vi "Read CAN FIFO Direct Dispatch.vi"(8 "error in (no error)":errorcluster, 9 "Timeout (ms)":i32, 11 "CIFTag in":refnum<class "CIFChannels.lvclass">) -> (0 "error out":errorcluster, 1 "timed out?":bool, 2 "Data":T1[](array[typedef]) {"Tags" format="%.0x"; "payload" format="%x"; "identifier" format="%x"}, 3 "CIFTag out":refnum<class "CIF_NIChn_FifoCAN.lvclass">, 4 "Header":T2)   [LabVIEW 2021, in "CIF_NIChn_FifoCAN.lvclass"]
uses:
  CIF_NIChn_FifoCAN.lvclass
  CIF_NIChn_FifoCAN.lvclass/CIF_NIChn_FifoCAN.ctl
  CIFChannels/Typedef/Direction.ctl
  CIFChannels/CIFChannels.lvclass
  CIFChannels/Typedef/Channel State.ctl
  NIChn/CIF_NIChn.lvclass
  D:/dev/CIF-LVCore/src/Channels/CIF_NIChn/NIChn/CIF_NIChn.lvclass
  D:/dev/CIF-LVCore/src/Channels/CIFChannels/CIFChannels.lvclass
  D:/dev/CIF-LVCore/src/Channels/CIF_NIChn/FIFO_CAN/CIF_NIChn_FifoCAN.lvclass
  <vilib>/CIFChannels/CIFChannelCore.lvlib
  ChannelRegistrar/typedef/Datatype CAN.ctl
  ChannelRegistrar/ChannelRegistrar.lvlib
  ChannelCommon/typedef/FIFO Header.ctl
  ChannelCommon/ChannelCommon.lvlib
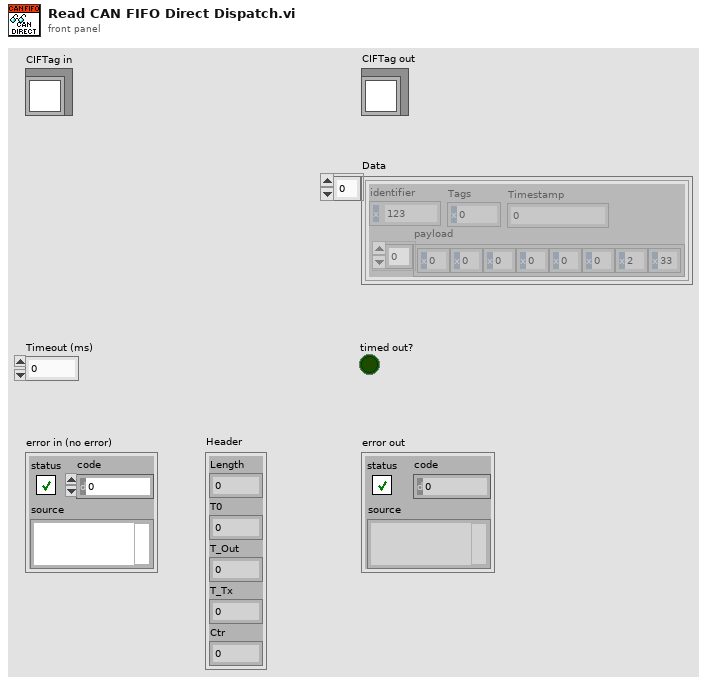
[diagram p1: front panel]
types:
  T1 = typedef "ChannelRegistrar.lvlib/Datatype CAN.ctl" = cluster{"payload":u8[], "identifier":u32, "Tags":u8, "Timestamp":u64}
  T2 = typedef "ChannelCommon.lvlib/FIFO Header.ctl" = cluster{"Length":u64, "T0":u64, "T_Out":u64, "T_Tx":u64, "Ctr":u64}
  T3 = typedef "CIFChannels.lvclass/Channel State.ctl" = enum16{"Creating", "Disconnected", "Connecting", "Connected", "Destroyed"}
  T4 = typedef "CIFChannels.lvclass/Direction.ctl" = enum16{"Publisher", "Subscriber"}
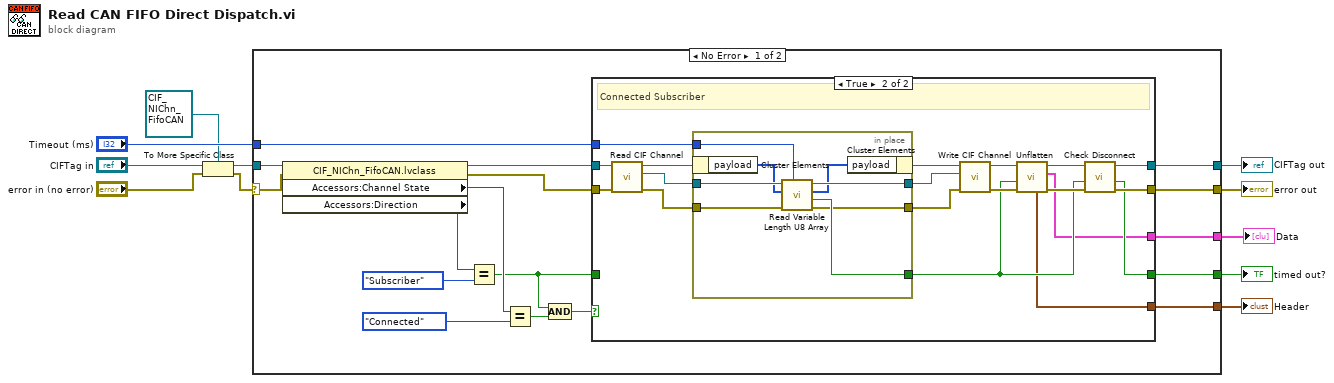
[diagram p0: block diagram]
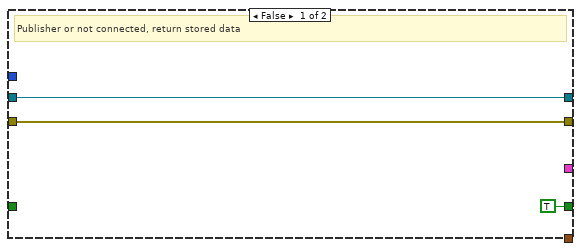
[diagram p2: hidden frame]
diagram:
  n1 = To More Specific Class(target class=refnum<class "CIF_NIChn_FifoCAN.lvclass"> refnum ("CIFTag in"), reference="CIFTag in", error in="error in (no error)") -> (specific class reference=w4:refnum<class "CIF_NIChn_FifoCAN.lvclass">, error out=w3:errorcluster)
  n2 = case shown="No Error" w3 {
    selector: w3 -> [w25 w60]
    tunnel: [w14 w60] -> w11
    tunnel: [w15 w59] -> w10
    tunnel: w4 -> [w26 w59]
    tunnel: [w28 _] -> w9
    tunnel: [w27 _] -> w1
    tunnel: "Timeout (ms)" -> [w13 _]
    tunnel: [w12 _] -> w7
    frame No Error {
      n3 = property class="CIF_NIChn_FifoCAN.lvclass"(reference=w26, error in=w25) -> (reference out=w24:refnum<class "CIF_NIChn_FifoCAN.lvclass">, error out=w23:errorcluster, "Accessors:Channel State"=w20:T3, "Accessors:Direction"=w22:T4)
      n4 = Equal?(x=w22, y=Direction."Subscriber") -> (x = y?=w16:bool)
      n5 = Equal?(x=w20, y=Channel_State."Connected") -> (x = y?=w18:bool)
      n6 = Compound Arithmetic op=AND(w16, w18) -> (w17:bool)
      n7 = case shown="True" w17 {
        tunnel: [TRUE ("timeout out") w40] -> w28
        tunnel: [_ w33] -> w27
        tunnel: w23 -> [w30 w49]
        tunnel: w24 -> [w31 w50]
        tunnel: w16 -> [_ _]
        tunnel: [w31 w48] -> w15
        tunnel: [w30 w47] -> w14
        tunnel: w13 -> [_ w39]
        tunnel: [_ w32] -> w12
        frame False {
          # "Publisher or not connected, return stored data"
        }
        frame True {
          # "Connected Subscriber"
          n8 = call "Read CIF Channel.vi"("error in (no error)"=w49, "CIFTag in"=w50) -> ("error out"=w44:errorcluster, "CIF Channel"=w45:refnum<k21>, "CIFTag out"=w46:refnum<class "CIF_NIChn_FifoCAN.lvclass">)  [unwired: 7 in]
          n9 = in-place {
            in-place-border: [w56] -> w34
            in-place-border: w45 -> [w58]
            in-place-border: w44 -> [w57]
            in-place-border: [w55] -> w41
            in-place-border: [w54] -> w42
            in-place-border: w39 -> [w53]
            n10 = in-place-cluster #1(w46) -> ("payload"=w52:u8[])
            n11 = call <vilib>:"Read Variable Length U8 Array.vi"("Timeout (ms)"=w53, "error in"=w57, "Payload in"=w52, "CIF Channel in"=w58) -> ("error out"=w54:errorcluster, "Timed out?"=w56:bool, "Payload out"=w51:u8[], "CIF Channel out"=w55:refnum<k21>)  [unwired: 4 in]
            n12 = in-place-cluster #1("payload"=w51) -> (w43:refnum<class "CIF_NIChn_FifoCAN.lvclass">)
          }
          n13 = call "Write CIF Channel.vi"("error in (no error)"=w42, "CIF Channel"=w41, "CIFTag in"=w43) -> ("error out"=w37:errorcluster, "CIFTag out"=w38:refnum<class "CIF_NIChn_FifoCAN.lvclass">)  [unwired: 7 in]
          n14 = call "Unflatten.vi"("error in (no error)"=w37, "timeout in"=w34, "CIFFifoCAN in"=w38) -> ("error out"=w35:errorcluster, "Data"=w33:T1[], "CIFFifoCAN out"=w36:refnum<class "CIF_NIChn_FifoCAN.lvclass">, "Header"=w32:T2)  [unwired: 5 in]
          n15 = call "Check Disconnect.vi"("error in (no error)"=w35, "timeout in"=w34, "CIFTag in"=w36) -> ("error out"=w47:errorcluster, "timeout out"=w40:bool, "CIFTag out"=w48:refnum<class "CIF_NIChn_FifoCAN.lvclass">)  [unwired: 5 in, 1 out]
        }
      }
    }
    frame Error {
    }
  }
  "error out" <- w11
  "CIFTag out" <- w10
  "timed out?" <- w9
  "Header" <- w7
  "Data" <- w1
